vi "TCP Send Receive.vi"(6 "timeout ms (1000)":i32=1000, 8 "error in (no error)":errorcluster caption="错误输入（无错误）", 9 "access (read/write)":enum16{"read/write", "read only", "write only"}(ring) caption="权限(read/write)", 10 "Data In":string caption="数据输入", 11 "connection ID":refnum<k5> caption="连接ID") -> (0 "error out":errorcluster caption="错误输出", 2 "Data Out":string caption="数据输出", 3 "connection ID Out":refnum<k5> caption="连接ID输出")   [LabVIEW 2020]
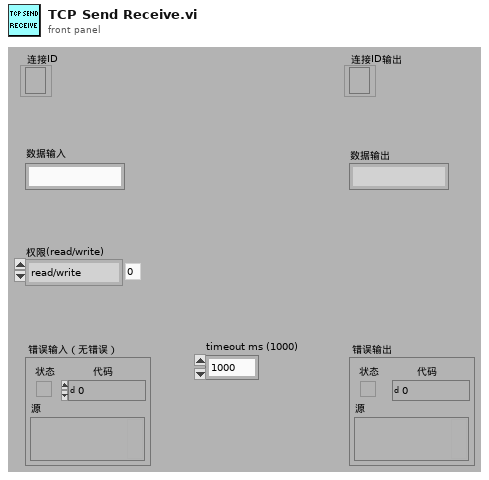
[diagram p1: front panel]
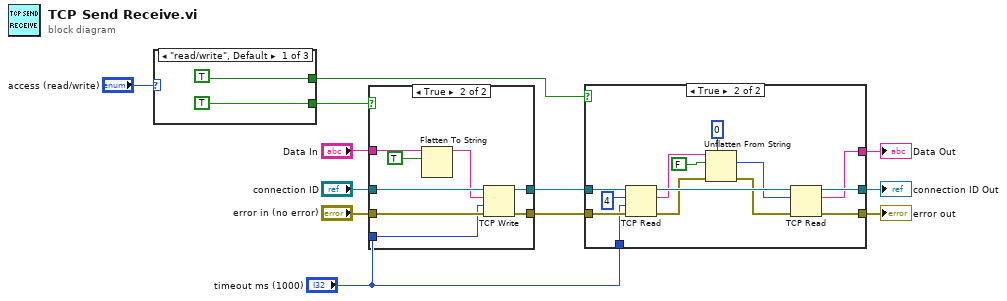
[diagram p0: block diagram]
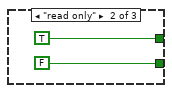
[diagram p2: hidden frame]
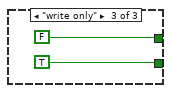
[diagram p3: hidden frame]
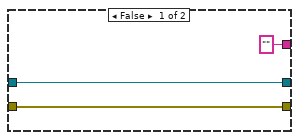
[diagram p4: hidden frame]
diagram:
  n1 = case shown="\"read/write\", Default" "access (read/write)" {
    tunnel: [TRUE FALSE TRUE] -> w3
    tunnel: [TRUE TRUE FALSE] -> w2
    frame "read/write", Default {
    }
    frame "read only" {
    }
    frame "write only" {
    }
  }
  n2 = case shown="True" w3 {
    tunnel: [w20 w28] -> w12
    tunnel: [w19 w27] -> w11
    tunnel: "connection ID" -> [w20 w26]
    tunnel: "error in (no error)" -> [w19 w25]
    tunnel: "Data In" -> [_ w24]
    tunnel: "timeout ms (1000)" -> [_ w21]
    frame False {
    }
    frame True {
      n3 = Flatten To String(anything=w24, prepend array or string size? (T)=TRUE) -> (data string=w22:string)  [unwired: 1 in, 3 out]
      n4 = TCP Write(connection ID=w26, data in=w22, error in (no error)=w25, 9:w21) -> (connection ID out=w28:refnum<k5>, error out=w27:errorcluster)  [unwired: 1 out]
    }
  }
  n5 = case shown="True" w2 {
    tunnel: w12 -> [w31 w45]
    tunnel: w11 -> [w30 w44]
    tunnel: [w31 w43] -> w10
    tunnel: [w30 w42] -> w9
    tunnel: ["" ("data out") w39] -> w5
    tunnel: "timeout ms (1000)" -> [_ w32]
    frame False {
    }
    frame True {
      n6 = TCP Read(connection ID=w45, bytes to read=4, error in (no error)=w44, 9:w32) -> (connection ID out=w40:refnum<k5>, data out=w37:string, error out=w35:errorcluster)  [unwired: 1 out]
      n7 = Unflatten From String(type=0, binary string=w37, data includes array or string size? (T)=FALSE, error in (no error)=w35) -> (value=w33:i32, error out=w34:errorcluster)  [unwired: 2 out]
      n8 = TCP Read(connection ID=w40, bytes to read=w33, error in (no error)=w34) -> (connection ID out=w43:refnum<k5>, data out=w39:string, error out=w42:errorcluster)  [unwired: 2 out]
    }
  }
  "Data Out" <- w5
  "error out" <- w9
  "connection ID Out" <- w10
